vi "CheckFileExist.vi"(0 "Path":string, 1 "error in (no error)":errorcluster) -> (2 "File Exists":bool, 3 "Overwrite File":bool, 4 "error out":errorcluster)   [LabVIEW 2011]
doc: "Checks whether the file to safe to already exists or not. If it exits, a user prompt is generate whether to overwrite this file or not."
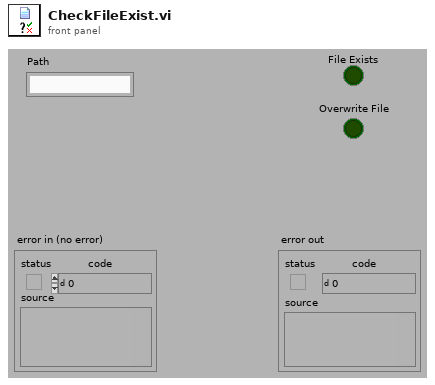
[diagram p1: front panel]
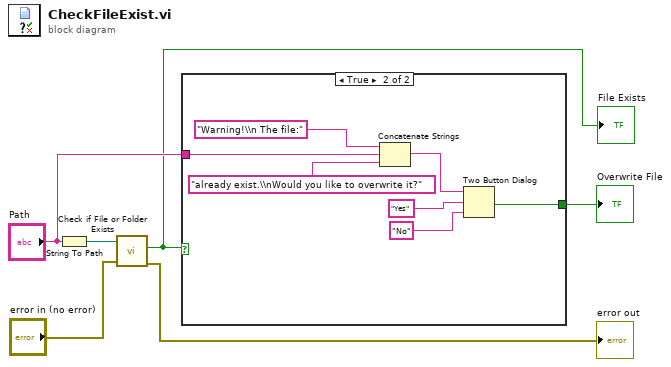
[diagram p0: block diagram]
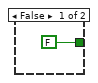
[diagram p2: hidden frame]
diagram:
  n1 = String To Path(string="Path") -> (path=w6:path)
  n2 = call <vilib>:"Check if File or Folder Exists.vi"("error in (no error)"="error in (no error)", "path"=w6) -> ("error out"=→"error out":errorcluster, "file or folder exists?"=w2:bool)  [unwired: 7 in, 1 out]
  "File Exists" <- w2
  n3 = case shown="True" w2 {
    tunnel: "Path" -> [_ w12]
    tunnel: [FALSE ("T button?") w8] -> w1
    frame False {
    }
    frame True {
      n4 = Concatenate Strings("Warning!\\n The file:", w12, "already exist.\\nWould you like to overwrite it?") -> (w11:string)
      n5 = Two Button Dialog(message=w11, 1:"No" ("Right Button Text (\"Cancel\")"), 2:"Yes" ("Right Button Text (\"Cancel\")")) -> (T button?=w8:bool)
    }
  }
  "Overwrite File" <- w1
